vi "Multiple Pin Multiple Session Query Context to Channel List.vi"(0 "Multiple Pin Multiple Sessions Query Context":refnum<class "MultiplePinMultipleSessionQueryContext.lvclass">, 5 "Expanded Pin Information":T1[](array[typedef]), 9 "Site Numbers In":i32[](array[numeric]), 11 "error in":errorcluster) -> (4 "Per-Session Channel List":string[](array[string]), 10 "Site Numbers Out":i32[](array[numeric]), 15 "error out":errorcluster)   [LabVIEW 2019]
uses:
  TSM Expanded Pin Information.ctl
  TSM Pin Type Identifier.ctl
  <vilib>/NI_TestStand_SemiconductorModule/NI_TestStand_Semiconductor_Module.lvlibp/PinMap/PinQueryContext/MultiplePinMultipleSessionQueryContext/MultiplePinMultipleSessionQueryContext.lvclass
  <vilib>/NI_TestStand_SemiconductorModule/NI_TestStand_Semiconductor_Module.lvlibp/PinMap/Advanced/GetPinsInPinGroups.vi
  <vilib>/NI_TestStand_SemiconductorModule/NI_TestStand_Semiconductor_Module.lvlibp
  <vilib>/NI_TestStand_SemiconductorModule/NI_TestStand_Semiconductor_Module.lvlibp/PinMap/PinQueryContext/PinQueryContext.lvclass
  C:/Program Files/National Instruments/LabVIEW 2019/vi.lib/NI_TestStand_SemiconductorModule/NI_TestStand_Semiconductor_Module.lvlibp/PinMap/PinQueryContext/PinQueryContext.lvclass
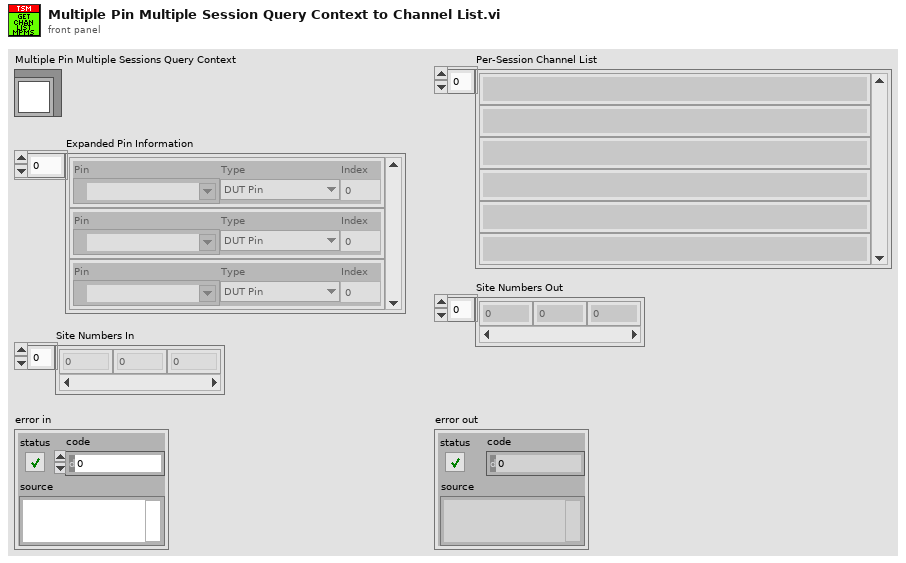
[diagram p1: front panel]
types:
  T1 = typedef "TSM Expanded Pin Information.ctl" = cluster{"Pin":tag, "Type":T2, "Index":i32}
  T2 = typedef "TSM Pin Type Identifier.ctl" = enum8{"DUT Pin", "System Pin", "Pin Group", "Not Determined"}
  T3 = typedef "NI_TestStand_Semiconductor_Module.lvlibp/SemiconductorModuleContext.ctl" = refnum<k7>
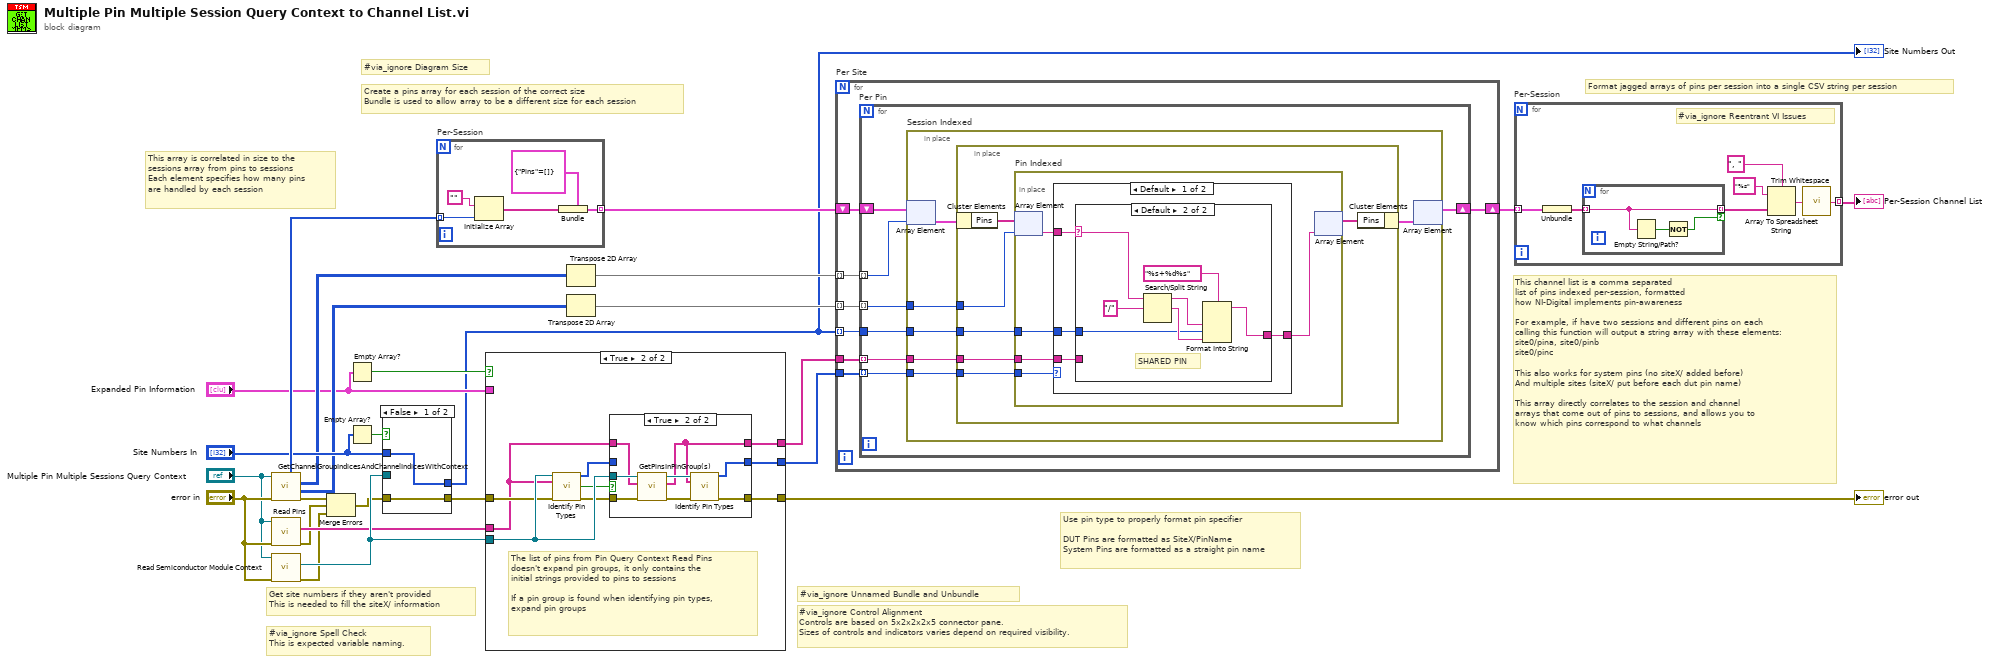
[diagram p0: block diagram]
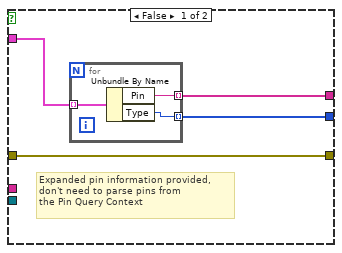
[diagram p2: hidden frame]
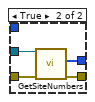
[diagram p4: hidden frame]
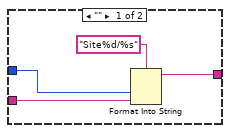
[diagram p5: hidden frame]
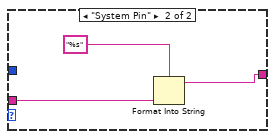
[diagram p6: hidden frame]
diagram:
  # "#via_ignore Unnamed Bundle and Unbundle"
  # "#via_ignore Diagram Size"
  # "#via_ignore Control Alignment\nControls are based on 5x2x2x2x5 connector pane.\nSizes of controls and indicators varies depend on required visibility."
  # "#via_ignore Spell Check\nThis is expected variable naming."
  # "Use pin type to properly format pin specifier\n\nDUT Pins are formatted as SiteX/PinName\nSystem Pins are formatted as a straight pin name"
  # "Create a pins array for each session of the correct size\nBundle is used to allow array to be a different size for each session"
  # "Format jagged arrays of pins per session into a single CSV string per session"
  # "This array is correlated in size to the \nsessions array from pins to sessions\nEach element specifies how many pins\nare handled by each session"
  # "Get site numbers if they aren't provided\nThis is needed to fill the siteX/ information"
  # "This channel list is a comma separated\nlist of pins indexed per-session, formatted\nhow NI-Digital implements pin-awareness\n\nFor example, if have two sessions and different pins on each\ncalling this function will output a string array with these elements:\nsite0/pina, site0/pinb\nsite0/pinc\n\nThis also works for system pins (no siteX/ added before)\nAnd multiple sites (siteX/ put before each dut pin name)\n\nThis array directly correlates to the session and channel \narrays that come out of pins to sessions, and allows you to\nknow which pins correspond to what channels"
  n1 = call <vilib>:"GetChannelGroupIndicesAndChannelIndicesWithContext.vi"("error in (no error)"="error in", "Publish Token"="Multiple Pin Multiple Sessions Query Context") -> ("error out"=w19:errorcluster, "Channel Indices"=w14:i32[][], "Channel Group Indices"=w15:i32[][], "Number of Pins Per Channel Group"=w20:i32[])  [unwired: 5 in, 1 out]
  n2 = call-dynamic "Read Pins.vi"("error in (no error)"="error in", "Pin Query Context"="Multiple Pin Multiple Sessions Query Context") -> ("error out"=w3:errorcluster, "Pins"=w12:tag[])  [unwired: 7 in, 1 out]
  n3 = call <vilib>:"Read Semiconductor Module Context.vi"("error in (no error)"="error in", "Pin Query Context"="Multiple Pin Multiple Sessions Query Context") -> ("error out"=w2:errorcluster, "Semiconductor Module Context"=w16:T3)  [unwired: 7 in, 1 out]
  n4 = Merge Errors(w19, w3, w2) -> (w4:errorcluster)
  n5 = Empty Array?(array="Expanded Pin Information") -> (empty?=w8:bool)
  n6 = Empty Array?(array="Site Numbers In") -> (empty?=w18:bool)
  n7 = case shown="False" w18 {
    tunnel: w4 -> [w27 w31]
    tunnel: [w27 w30] -> w13
    tunnel: w16 -> [_ w29]
    tunnel: [w26 w28] -> w6
    tunnel: "Site Numbers In" -> [w26 _]
    frame False {
    }
    frame True {
      n8 = call <vilib>:"GetSiteNumbers.vi"("error in (no error)"=w31, "Semiconductor Module Context"=w29) -> ("error out"=w30:errorcluster, "Site Numbers"=w28:i32[])  [unwired: 6 in, 2 out]
    }
  }
  "Site Numbers Out" <- w6
  n9 = for "Per-Session" {
    tunnel: w20 -> [w35] mode=indexing
    tunnel: [w33] -> w23 mode=indexing
    n10 = Initialize Array("", w35) -> (w34:string[])
    n11 = Bundle(cluster=cluster{"Pins":string[]} {"Pins"=[]}, "Pins"=w34) -> (w33:cluster{"Pins":string[]})
  }
  n12 = case shown="True" w8 {
    tunnel: w16 -> [_ w52]
    tunnel: w13 -> [w37 w51]
    tunnel: w12 -> [_ w47]
    tunnel: [w39 w46] -> w11
    tunnel: [w38 w45] -> w10
    tunnel: [w37 w44] -> w9
    tunnel: "Expanded Pin Information" -> [w40 _]
    frame False {
      # "Expanded pin information provided, \ndon't need to parse pins from \nthe Pin Query Context"
      n13 = for {
        tunnel: w40 -> [w43] mode=indexing
        tunnel: [w42] -> w39 mode=indexing
        tunnel: [w41] -> w38 mode=indexing
        n14 = Unbundle By Name(w43) -> ("Pin"=w42:tag, "Type"=w41:T2)
      }
    }
    frame True {
      # "The list of pins from Pin Query Context Read Pins\ndoesn't expand pin groups, it only contains the \ninitial strings provided to pins to sessions\n\nIf a pin group is found when identifying pin types, \nexpand pin groups"
      n15 = call "Identify Pin Types.vi"("TSM context"=w52, "Pins and/or Pin Groups"=w47, "error in"=w51) -> ("Pin Types"=w48:T2[], "Pin Group Found?"=w50:bool, "error out"=w49:errorcluster)  [unwired: 10 in]
      n16 = case shown="True" w50 {
        tunnel: w52 -> [_ w63]
        tunnel: w49 -> [w53 w57]
        tunnel: w48 -> [w55 _]
        tunnel: w47 -> [w54 w60]
        tunnel: [w55 w59] -> w45
        tunnel: [w54 w58] -> w46
        tunnel: [w53 w56] -> w44
        frame False {
        }
        frame True {
          n17 = call-poly <vilib>:"GetPinsInPinGroup(s).vi"("error in (no error)"=w57, "Pin Groups"=w60, "Semiconductor Module Context"=w63) -> ("error out"=w61:errorcluster, "Pins"=w58:tag[], "Semiconductor Module Context Out"=w62:T3)  [unwired: 6 in]
          n18 = call "Identify Pin Types.vi"("TSM context"=w62, "Pins and/or Pin Groups"=w58, "error in"=w61) -> ("Pin Types"=w59:T2[], "error out"=w56:errorcluster)  [unwired: 10 in, 1 out]
        }
      }
    }
  }
  "error out" <- w9
  n19 = Transpose 2D Array(2D array=w15) -> (transposed array=w25:i32[][])
  n20 = Transpose 2D Array(2D array=w14) -> (transposed array=w24:i32[][])
  n21 = for "Per Site" {
    tunnel: w25 -> [w70] mode=indexing
    tunnel: w24 -> [w69] mode=indexing
    shift-right: [w67] -> w22
    shift-left: w23 -> [w68]
    tunnel: w11 -> [w66]
    tunnel: w6 -> [w65] mode=indexing
    tunnel: w10 -> [w64]
    n22 = for "Per Pin" {
      tunnel: w70 -> [w76] mode=indexing
      tunnel: w69 -> [w75] mode=indexing
      shift-right: [w74] -> w67
      shift-left: w68 -> [w77]
      tunnel: w66 -> [w73] mode=indexing
      tunnel: w65 -> [w72]
      tunnel: w64 -> [w71] mode=indexing
      n23 = in-place "Session Indexed" {
        in-place-border: w75 -> [w82]
        in-place-border: w73 -> [w81]
        in-place-border: w72 -> [w79]
        in-place-border: w71 -> [w78]
        n24 = in-place-array #1(w77, w76) -> (w83:cluster{"Pins":string[]})
        n25 = in-place {
          in-place-border: w82 -> [w88]
          in-place-border: w81 -> [w87]
          in-place-border: w79 -> [w85]
          in-place-border: w78 -> [w84]
          n26 = in-place-cluster #2(w83) -> ("Pins"=w89:string[])
          n27 = in-place "Pin Indexed" {
            in-place-border: w87 -> [w94]
            in-place-border: w85 -> [w93]
            in-place-border: w84 -> [w91]
            n28 = in-place-array #3(w89, w88) -> (w90:string)
            n29 = case shown="Default" w91 {
              tunnel: w94 -> [w98 w112]
              tunnel: w93 -> [w97 _]
              tunnel: [w96 w111] -> w92
              tunnel: w90 -> [w95 _]
              frame Default {
                n30 = case shown="Default" w95 {
                  selector: w95 -> [_ w109]
                  tunnel: w98 -> [w102 _]
                  tunnel: w97 -> [w101 w105]
                  tunnel: [w100 w104] -> w96
                  frame "" {
                    n31 = Format Into String(format string="Site%d/%s", w101, w102) -> (resulting string=w100:string)  [unwired: 2 in, 1 out]
                  }
                  frame Default {
                    # "SHARED PIN"
                    n32 = Search/Split String(string=w109, search string/char (-)="/") -> (substring before match=w107:string, match + rest of string=w106:string)  [unwired: 1 in, 1 out]
                    n33 = Format Into String(format string="%s+%d%s", w107, w105, w106) -> (resulting string=w104:string)  [unwired: 2 in, 1 out]
                  }
                }
              }
              frame "System Pin" {
                n34 = Format Into String(format string="%s", w112) -> (resulting string=w111:string)  [unwired: 2 in, 1 out]
              }
            }
            n35 = in-place-array #3(w92) -> (w86:string[])  [unwired: 1 out]
          }
          n36 = in-place-cluster #2("Pins"=w86) -> (w80:cluster{"Pins":string[]})
        }
        n37 = in-place-array #1(w80) -> (w74:cluster{"Pins":string[]}[])  [unwired: 1 out]
      }
    }
  }
  n38 = for "Per-Session" {
    tunnel: w22 -> [w119] mode=indexing
    tunnel: [w115] -> w21 mode=indexing
    # "#via_ignore Reentrant VI Issues"
    n39 = Unbundle(w119) -> ("Pins"=w114:string[])
    n40 = for {
      tunnel: w114 -> [w122] mode=indexing
      tunnel: [w122] -> w113 mode=indexing if=w120
      n41 = Empty String/Path?(string/path=w122) -> (empty?=w121:bool)
      n42 = Not(x=w121) -> (.not. x?=w120:bool)
    }
    n43 = Array To Spreadsheet String(delimiter (Tab)=", ", array=w113, 3:"%s" ("format string")) -> (spreadsheet string=w116:string)
    n44 = call <vilib>:"Trim Whitespace.vi"("string"=w116) -> ("trimmed string"=w115:string)  [unwired: 1 in]
  }
  "Per-Session Channel List" <- w21
